vi "TestStand, Set Step Data.vi"(6 "TS index":i32, 8 "error in":errorcluster, 10 "Result":dbl=nan format="%.5f", 11 "Sequence Context":refnum<k7>) -> (0 "error out":errorcluster, 3 "Sequence Context Out":refnum<k7>)   [LabVIEW 2010]
doc: "Transfers measurement results to the default TestStand Multiple Numeric Test data array (RunState.Step.NumericArray)."
uses:
  <vilib>/addons/TestStand/_TSUtility.llb/TestStand - Set Property Value (Number).vi
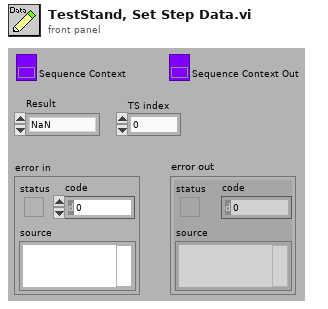
[diagram p1: front panel]
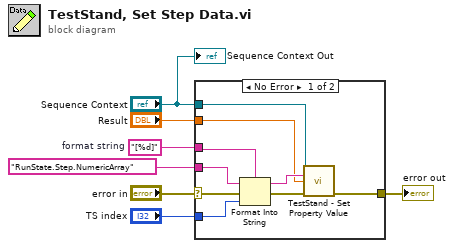
[diagram p0: block diagram]
diagram:
  w5 = "[%d]"  # format string
  n1 = case shown="No Error" "error in" {
    selector: "error in" -> [w16 w17]
    tunnel: [w13 w17] -> w7
    tunnel: "Sequence Context" -> [w14 _]
    tunnel: w5 -> [w15 _]
    tunnel: "RunState.Step.NumericArray" ("suffix") -> [w12 _]
    tunnel: "Result" -> [w9 _]
    tunnel: "TS index" -> [w8 _]
    frame No Error {
      n2 = Format Into String(format string=w15, initial string=w12, error in=w16, w8) -> (resulting string=w11:string, error out=w10:errorcluster)
      n3 = call-poly <vilib>:"TestStand - Set Property Value.vi"("Sequence Context In"=w14, "Lookup String"=w11, "New Value"=w9, "error in (no error)"=w10) -> ("error out"=w13:errorcluster)  [unwired: 10 in, 1 out]
    }
    frame Error {
    }
  }
  "error out" <- w7
  "Sequence Context Out" <- "Sequence Context"
